vi "TW Edit - Stage 1.vi"(6 "Channels to Create":T2[](array[typedef]), 8 "error in":errorcluster, 9 "Icon Overlay":T1={"Text"="", "Background color"=7208704, "Text color"=0}, 10 "New Subname":string, 11 "Template Project Path":path) -> (0 "error out":errorcluster)   [LabVIEW 2021, in "Plugin Generator.lvlib"]
uses:
  Plugin Generator.lvlib
  <vilib>/CIF Foundation/CIF Core/Channels/ChannelRegistrar/typedef/Channel Definition for Scripting.ctl
  <vilib>/CIF Foundation/CIF Channels Core/CIFChannels/Typedef/Direction.ctl
  <vilib>/CIF Foundation/CIF Core/Channels/ChannelRegistrar/typedef/Registered Channel Types.ctl
  <vilib>/CIF Foundation/CIF LabVIEW Scripting/LV Scripting/Typedef/Icon Overlay.ctl
  <vilib>/CIF Foundation/CIF LabVIEW Scripting/LV Scripting/LV Scripting Utilities.lvlib
  <vilib>/CIF Foundation/CIF Channels Core/CIFChannels/CIFChannels.lvclass
  <vilib>/CIF Foundation/CIF Core/Channels/ChannelRegistrar/ChannelRegistrar.lvlib
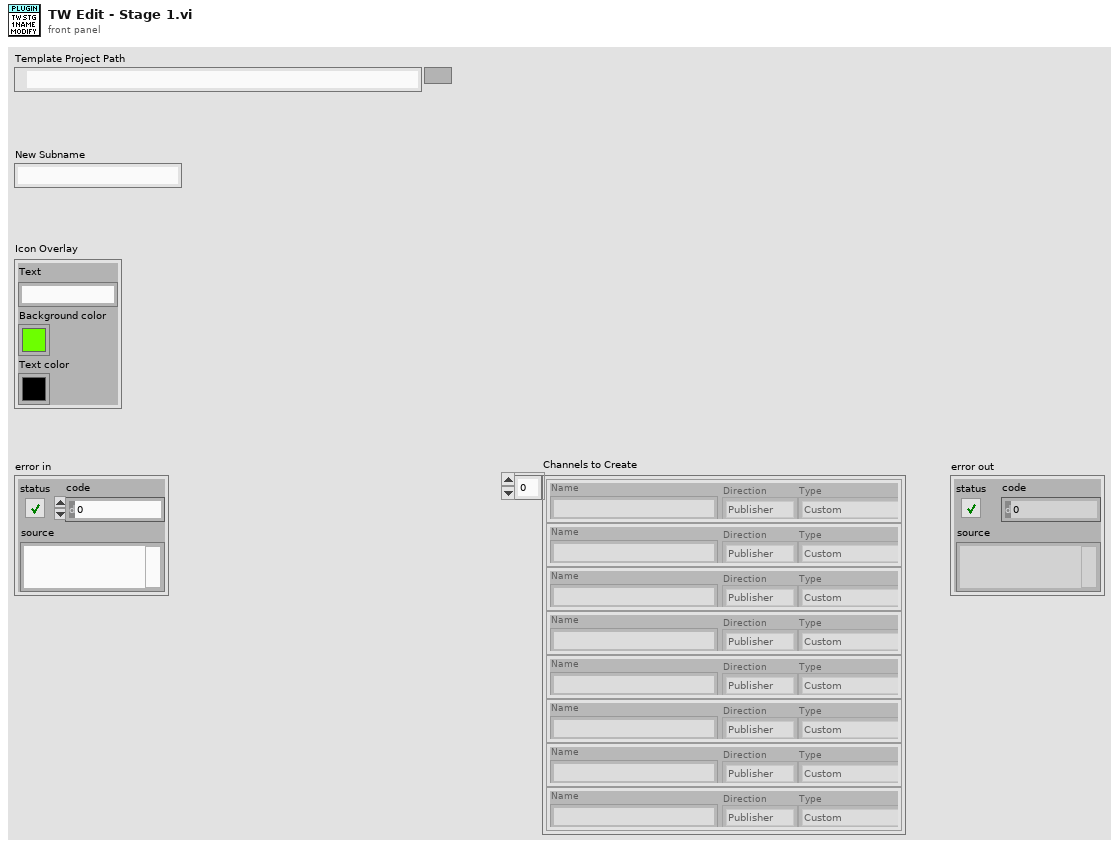
[diagram p1: front panel]
types:
  T1 = typedef "LV Scripting Utilities.lvlib/Icon Overlay.ctl" = cluster{"Text":string, "Background color":u32, "Text color":u32}
  T2 = typedef "ChannelRegistrar.lvlib/Channel Definition for Scripting.ctl" = cluster{"Name":string, "Direction":T3, "Type":T4}
  T3 = typedef "CIFChannels.lvclass/Direction.ctl" = enum16{"Publisher", "Subscriber"}
  T4 = typedef "ChannelRegistrar.lvlib/Registered Channel Types.ctl" = enum16{"Custom", "Double_Tag", "I64_Tag", "U64_Tag", "U8_FIFO", "CAN_FIFO", "L2Enet_FIFO", "DAQ_FIFO", "Universal_FIFO", "String_Tag"}
  T5 = cluster{"Library Name":string, "Update Folder Name":bool}[]
  T6 = typedef "LV Scripting Utilities.lvlib/Target References.ctl" = cluster{"Target Reference":refnum<vi>, "VI References":refnum<vi>[], "Library References":refnum<vi>[], "Build References":refnum<vi>[]}
  T7 = typedef "LV Scripting Utilities.lvlib/Library Map.ctl" = map{string, refnum<vi>}
  T8 = typedef "LV Scripting Utilities.lvlib/VI Map.ctl" = map{string, refnum<vi>}
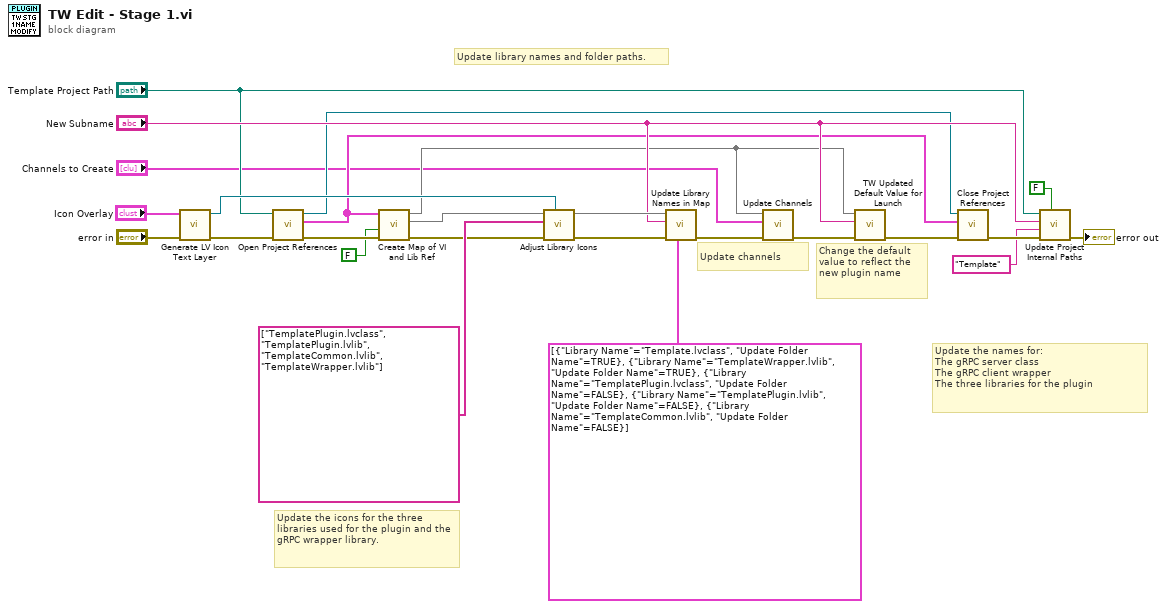
[diagram p0: block diagram]
diagram:
  # "Update channels"
  # "Update library names and folder paths."
  # "Change the default value to reflect the new plugin name"
  # "Update the names for:\nThe gRPC server class\nThe gRPC client wrapper\nThe three libraries for the plugin"
  # "Update the icons for the three libraries used for the plugin and the gRPC wrapper library."
  n1 = call <vilib>:"Generate LV Icon Text Layer.vi"("error in (no error)"="error in", "Icon Overlay"="Icon Overlay") -> ("error out"=w14:errorcluster, "Icon.lvlclass out"=w21:refnum<class "Icon.lvclass">)  [unwired: 7 in, 1 out]
  n2 = call <vilib>:"Open Project References.vi"("error in"=w14, "Project Path"="Template Project Path") -> ("error out"=w13:errorcluster, "VI, Library, and Build References"=w10:T6[], "Project Reference"=w11:refnum<vi>)  [unwired: 7 in]
  n3 = call <vilib>:"Create Map of VI and Lib Ref.vi"("error in"=w13, "RT Target"=FALSE, "VI, Library, and Build References"=w10) -> ("error out"=w20:errorcluster, "Library Map"=w22:T7, "VI Map"=w5:T8)  [unwired: 5 in, 1 out]
  n4 = call <vilib>:"Adjust Library Icons.vi"("Overlay Icon"=w21, "error in"=w20, "Library Names"=string[] ["TemplatePlugin.lvclass", "TemplatePlugin.lvlib", "TemplateCommon.lvlib", "TemplateWrapper.lvlib"], "Library Map in"=w22) -> ("error out"=w6:errorcluster, "Library Map out"=w19:map{string, refnum<vi>})  [unwired: 5 in, 1 out]
  n5 = call <vilib>:"Update Library Names in Map.vi"("Libraries"=T5 [{"Library Name"="Template.lvclass", "Update Folder Name"=TRUE}, {"Library Name"="TemplateWrapper.lvlib", "Update Folder Name"=TRUE}, {"Library Name"="TemplatePlugin.lvclass", "Update Folder Name"=FALSE}, {"Library Name"="TemplatePlugin.lvlib", "Update Folder Name"=FALSE}, {"Library Name"="TemplateCommon.lvlib", "Update Folder Name"=FALSE}], "error in"=w6, "New Subname"="New Subname", "Library Map"=w19) -> ("error out"=w4:errorcluster)  [unwired: 6 in, 1 out]
  n6 = call "Update Channels.vi"("error in"=w4, "Channels to Create"="Channels to Create", "VI Map"=w5) -> ("error out"=w3:errorcluster)  [unwired: 8 in]
  n7 = call "TW Updated Default Value for Launch.vi"("error in"=w3, "New Subname"="New Subname", "Name to VI Map"=w5) -> ("error out"=w12:errorcluster)  [unwired: 8 in]
  n8 = call <vilib>:"Close Project References.vi"("error in"=w12, "VI, Library, and Build References"=w10, "Project Reference"=w11) -> ("error out"=w9:errorcluster)  [unwired: 8 in]
  n9 = call <vilib>:"Update Project Internal Paths.vi"("Rename Project"=FALSE, "error in (no error)"=w9, "Replace Subname"="Template", "New Subname"="New Subname", "Project Path"="Template Project Path") -> ("error out"=→"error out":errorcluster)  [unwired: 6 in]
